vi "CreatePublicEvents.vi"(8 "error in (no error)":errorcluster, 11 "Instrument.AFM_DLog in":refnum<class "Instrument.AFM_DLog.lvclass">) -> (0 "error out":errorcluster, 3 "Instrument.AFM_DLog out":refnum<class "Instrument.AFM_DLog.lvclass">)   [LabVIEW 2019]
uses:
  <userlib>/LevyLab/RemoteControl/RemoteControl/Typedefs/Message--Cluster.ctl
  <userlib>/LevyLab/RemoteControl/RemoteControl/RemoteControl.lvclass
  Typedefs/PublicEvents--AFM_DLog.MessageFromProcess.ctl
  Instrument.AFM_DLog.lvclass
  C:/Program Files (x86)/National Instruments/LabVIEW 2019/user.lib/LevyLab/Instrument Framework/Instrument Types/SCPI/Instrument.SCPI.lvclass
  C:/Program Files (x86)/National Instruments/LabVIEW 2019/user.lib/LevyLab/Instrument Framework/Instrument/Instrument.lvclass
  C:/Program Files (x86)/National Instruments/LabVIEW 2019/vi.lib/JKI/JKI SMO/SMO/SMO.lvclass
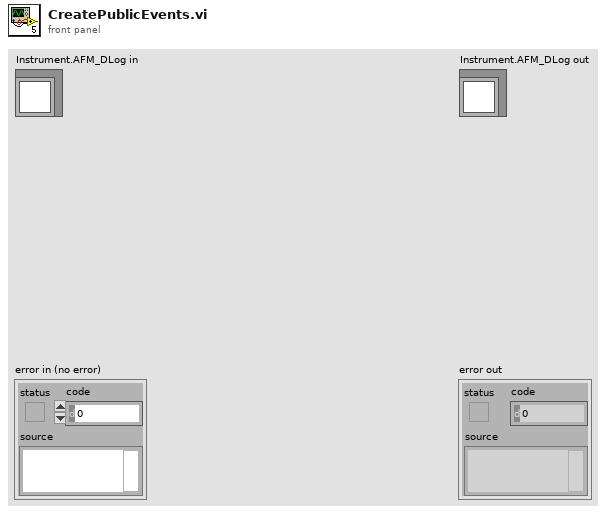
[diagram p1: front panel]
types:
  T1 = typedef "Instrument.AFM_DLog.lvclass/PublicEvents--AFM_DLog.MessageFromProcess.ctl" = cluster{"Message":T2}
  T2 = typedef "RemoteControl.lvlib/RemoteControl.lvclass/Message--Cluster.ctl" = cluster{"Command":string, "Data":variant, "ID":string}
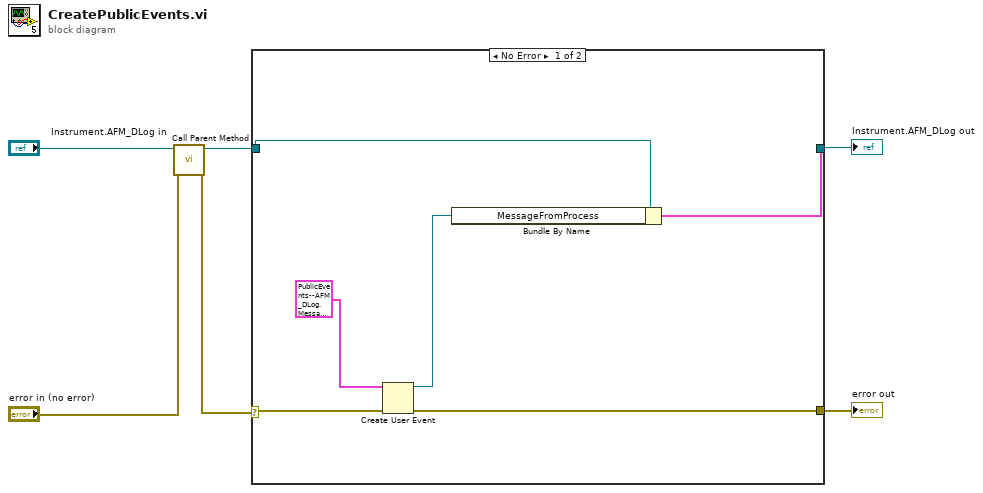
[diagram p0: block diagram]
diagram:
  n1 = call-parent "Call Parent Method"("error in (no error)"="error in (no error)", "Instrument"="Instrument.AFM_DLog in") -> ("error out"=w3:errorcluster, "Instrument out"=w1:refnum<class "Instrument.AFM_DLog.lvclass">)  [unwired: 8 in]
  n2 = case shown="No Error" w3 {
    selector: w3 -> [w10 w14]
    tunnel: [w8 w14] -> w5
    tunnel: [w11 w13] -> w6
    tunnel: w1 -> [w12 w13]
    frame No Error {
      n3 = Create User Event(user event datatype=T1 {"Message"={"Command"="", "Data"=variant(string ""), "ID"=""}} ("MessageFromProcess"), error in=w10) -> (user event=w9:refnum<user-event>, error out=w8:errorcluster)
      n4 = Bundle By Name(cluster=w12, "MessageFromProcess"=w9) -> (w11:cluster{})
    }
    frame Error {
    }
  }
  "error out" <- w5
  "Instrument.AFM_DLog out" <- w6
